vi "Main.vi"(10 "DAQ Type":enum16{"Hardware", "Simulation"}(ring), 11 "Module Admin":refnum<class "Delacor_lib_QMH_Module Admin.lvclass">) -> ()   [LabVIEW 2021, in "ARINC.lvlib"]
doc: "This template is based off of the Queued Message Handler design pattern and the Queued Message Handler project template that ships with LabVIEW.\n\nThe main difference is that the queue is private to this module and communication between modules is performed via Broadcast and Request events.\n\nRequest events are wrapped in public API methods and are handled in the Event Handling Loop (EHL) of this VI. Any module can register for Broadcast events sent by this module. The EHL generates messages based on user interface actions.\n\nThe Message Handling Loop (MHL) processes messages generated by the EHL, or by other messages. The messages are string values, so new messages can be added easily to the Message Cases case structure in the MHL. Each message cluster can also provide an optional value for Message Data, which is a variant that can be converted to whatever message-specific data is required.\n_____\nBased on DQMH Project Template 6.1.0.94."
uses:
  ARINC.lvlib
  <vilib>/Delacor/Delacor QMH/Libraries/Module Admin_class/Delacor_lib_QMH_Module Admin.lvclass
  Class/AIT 429/AIT 429.lvclass
  C:/repository/common_ATE/Libraries/ARINC/Class/Abstract/Abstract.lvclass
  Class/Abstract/Abstract.lvclass
  Module Data--cluster.ctl
  <vilib>/Delacor/Delacor QMH/Libraries/Message Queue_class/Delacor_lib_QMH_Message Queue.lvclass/Delacor_lib_QMH_Message Queue.ctl
  Stop Argument--cluster.ctl
  <vilib>/Delacor/Delacor QMH/Libraries/Module Admin_class/Delacor_lib_QMH_Module Admin.lvclass/Delacor_lib_QMH_Module Admin.ctl
  REQ Initialize Hardware Argument--cluster.ctl
  REQ Initialize Hardware (Reply Payload)--cluster.ctl
  REQ Close Ref Argument--cluster.ctl
  <vilib>/Utility/miscctls.llb/LVPointTypeDef.ctl
  <vilib>/Delacor/Delacor QMH/Libraries/Message Queue_class/Delacor_lib_QMH_Enqueue Message (Single).vi
  <vilib>/Delacor/Delacor QMH/Libraries/Module Admin_class/Delacor_lib_QMH_Get External Launch.vi
  <vilib>/Utility/error.llb/Error Cluster From Error Code.vi
  <vilib>/ErrorRing/Error Ring.xnode
  <vilib>/Delacor/Delacor QMH/Libraries/Message Queue_class/Delacor_lib_QMH_Message Queue.lvclass
panel:
  out "error out":errorcluster
  out "Status":string
  in  "Simulate MHL Error":bool
  in  "Simulate EHL Error":bool
  # "Other QMH Modules communicate with this Module via its Public API (wrappers for its Request Events).\n\nThis Module communicates with other Modules via its Broadcast Events.\nAny module that wants to get these messages, just registers for this module's Broadcast events."
  # "This template is for the Delacor Modified Queued Message Handler design pattern.\n\nSee the block diagram for more information on how to use this template."
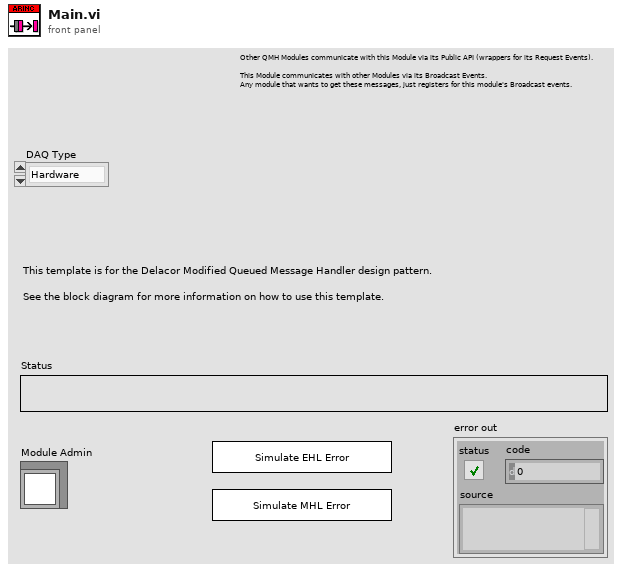
[diagram p1: front panel]
types:
  T1 = typedef "ARINC.lvlib/Request Events--cluster.ctl" = cluster{"Stop Module":refnum<user-event>, "Show Panel":refnum<user-event>, "Hide Panel":refnum<user-event>, "Get Module Execution Status":refnum<user-event>, "Show Diagram":refnum<user-event>, "REQ Initialize Hardware":refnum<user-event>, "REQ Close Ref":refnum<user-event>}
  T2 = typedef "ARINC.lvlib/Module Data--cluster.ctl" = cluster{"Status":string, "Abstract.lvclass":refnum<class "Abstract.lvclass">, "Connection Ref":variant}
  T3 = enum32{"invalid lock state", "Not Locked", "Locked (No Password)", "Password-protected"}
  T4 = typedef "ARINC.lvlib/Stop Argument--cluster.ctl" = cluster{"Origin":string, "Exit via Stop Module Req?":bool, "Wait for Module to stop?":bool}
  T5 = typedef "ARINC.lvlib/REQ Initialize Hardware Argument--cluster.ctl" = cluster{"Connection Ref":variant, "Wait Notifier":refnum<notifier>, "wait for reply":bool}
  T6 = typedef "ARINC.lvlib/REQ Close Ref Argument--cluster.ctl" = cluster{"Boolean":bool}
  T7 = typedef "LVPointTypeDef.ctl" = cluster{"Horizontal":i16, "Vertical":i16}
  T8 = enum32{"Invalid", "Standard", "Closed", "Hidden", "Minimized", "Maximized"}
  T9 = typedef "ARINC.lvlib/REQ Initialize Hardware (Reply Payload)--cluster.ctl" = cluster{"Connect?":bool, "error":errorcluster}
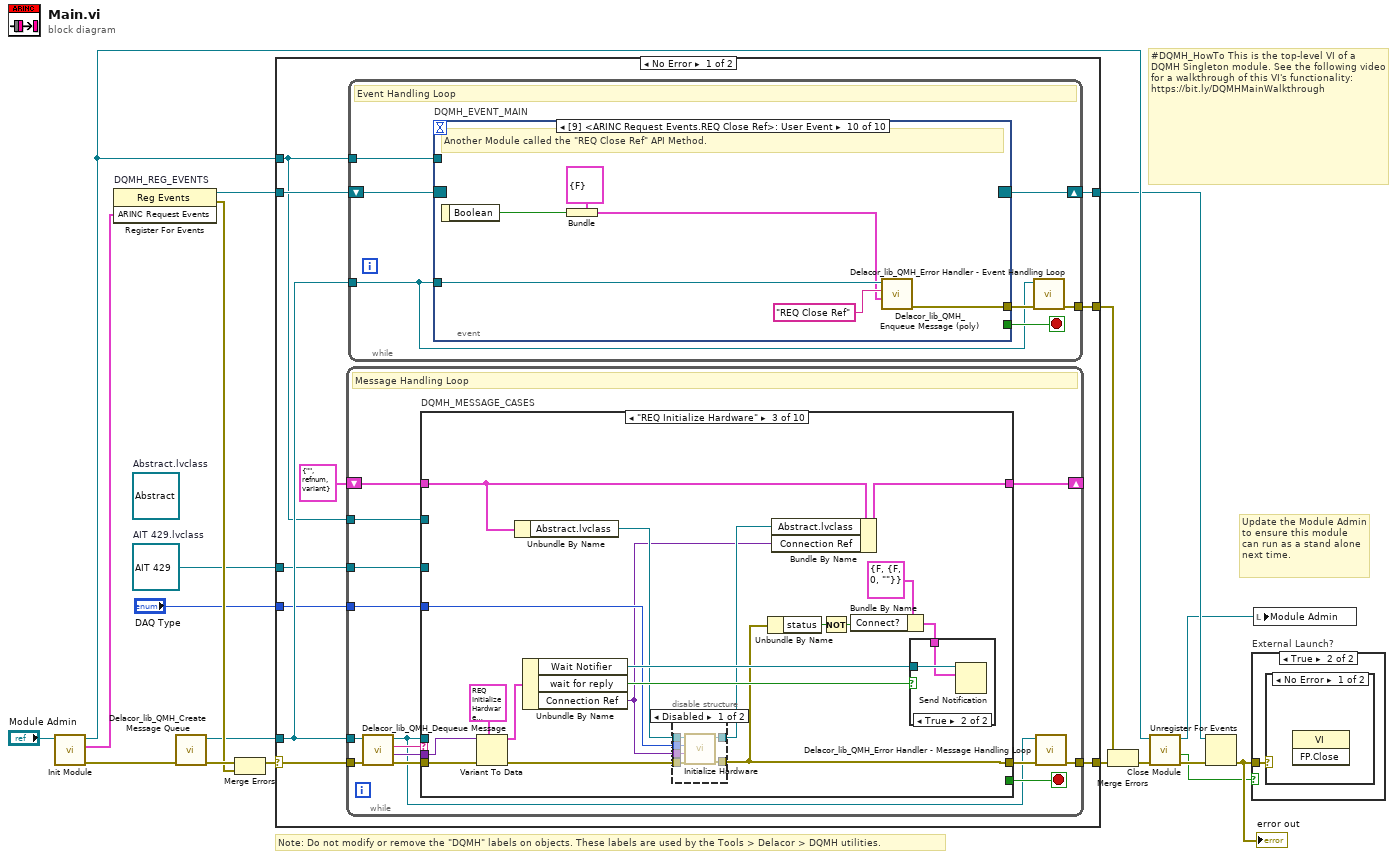
[diagram p0: block diagram]
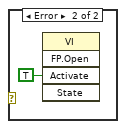
[diagram p3: hidden frame]
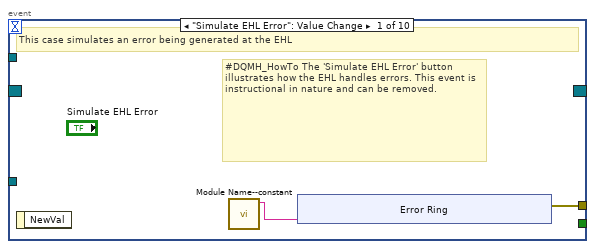
[diagram p4: hidden frame]
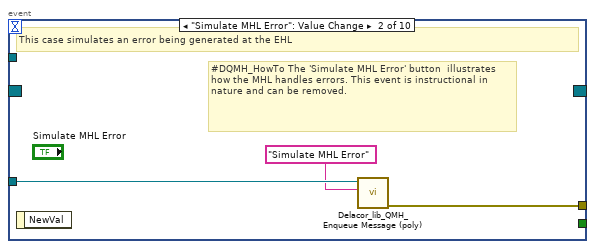
[diagram p5: hidden frame]
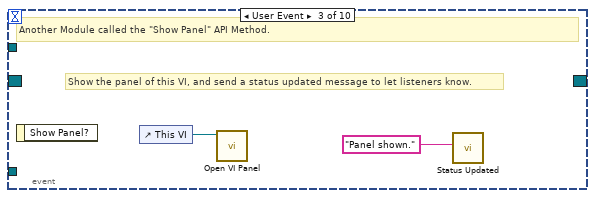
[diagram p6: hidden frame]
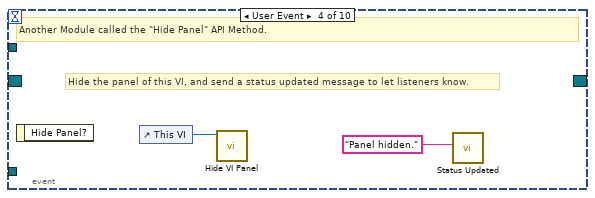
[diagram p7: hidden frame]
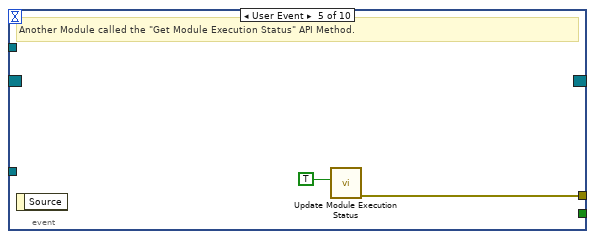
[diagram p8: hidden frame]
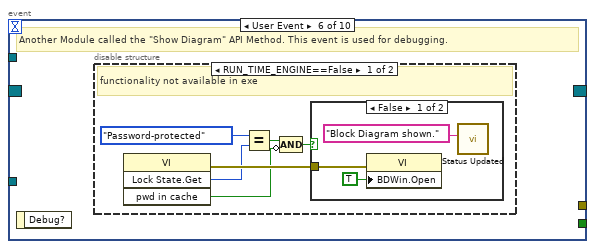
[diagram p9: hidden frame]
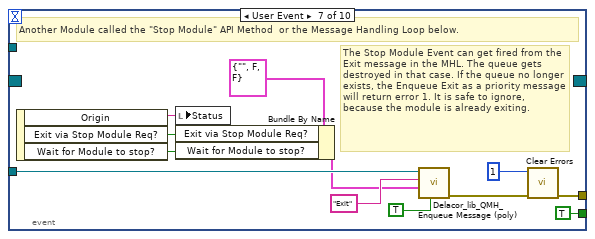
[diagram p12: hidden frame]
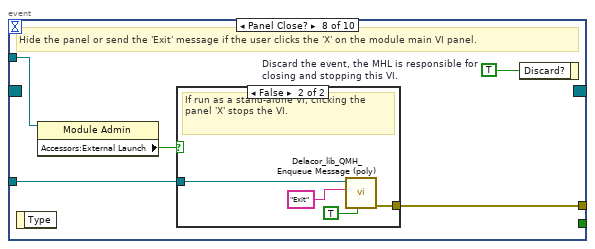
[diagram p13: hidden frame]
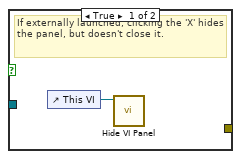
[diagram p14: hidden frame]
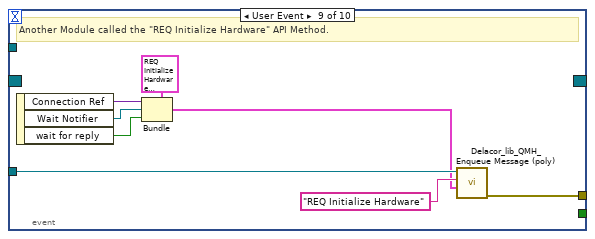
[diagram p15: hidden frame]
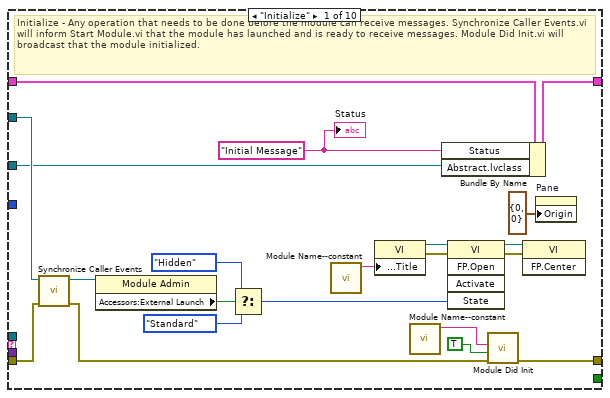
[diagram p16: hidden frame]
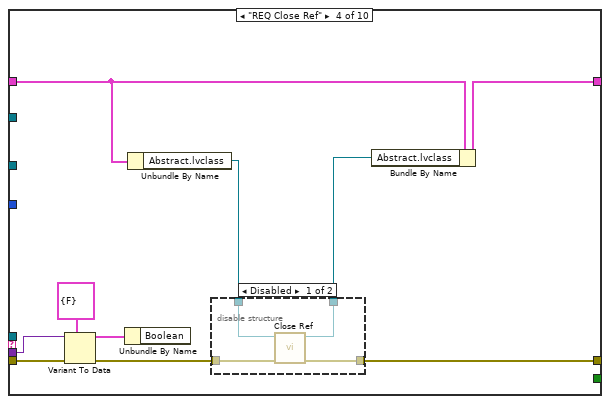
[diagram p20: hidden frame]
diagram:
  w2 = refnum<class "AIT 429.lvclass"> refnum  # AIT 429.lvclass
  (unwired) refnum<class "Abstract.lvclass"> refnum  # Abstract.lvclass
  # "#DQMH_HowTo This is the top-level VI of a DQMH Singleton module. See the following video for a walkthrough of this VI's functionality: https://bit.ly/DQMHMainWalkthrough"
  # "Note: Do not modify or remove the \"DQMH\" labels on objects. These labels are used by the Tools > Delacor > DQMH utilities."
  # "Update the Module Admin to ensure this module can run as a stand alone next time."
  n1 = call "Init Module.vi"("Singleton Module Admin in"="Module Admin") -> ("error out"=w18:errorcluster, "ARINC Request Events"=w7:T1, "Singleton Module Admin out"=w10:refnum<class "Delacor_lib_QMH_Module Admin.lvclass">)  [unwired: 8 in]
  n2 = register-events "DQMH_REG_EVENTS"(w7) -> (reference out=w8:refnum<event-registration>, error out=w11:errorcluster)  [unwired: 2 in]
  n3 = call <vilib>:"Delacor_lib_QMH_Create Message Queue.vi"("error in"=w18) -> ("error out"=w13:errorcluster, "Message Queue"=w6:refnum<class "Delacor_lib_QMH_Message Queue.lvclass">)  [unwired: 9 in]
  n4 = Merge Errors(w13, w11) -> (w12:errorcluster)
  n5 = case shown="No Error" w12 {
    selector: w12 -> [w27 w241]
    tunnel: [w29 w240] -> w19
    tunnel: [w26 w246] -> w9
    tunnel: w8 -> [w24 w246]
    tunnel: w6 -> [w23 w239]
    tunnel: [w28 _] -> w16
    tunnel: w10 -> [w22 w242]
    tunnel: w2 -> [w21 _]
    tunnel: "DAQ Type" -> [w20 _]
    frame No Error {
      n6 = while {
        tunnel: w23 -> [w104]
        shift-right: [w108] -> _
        shift-left: T2 {"Status"="", "Abstract.lvclass"=refnum, "Connection Ref"=variant} ("Data Cluster") -> [w109]
        tunnel: w27 -> [w112]
        tunnel: [w110] -> w29
        tunnel: w22 -> [w102]
        tunnel: w21 -> [w101]
        tunnel: w20 -> [w100]
        stop <- w107 stop-if-true
        # "Message Handling Loop"
        n7 = call-dynamic "Delacor_lib_QMH_Dequeue Message.vi"("error in"=w112, "Message Queue in"=w104) -> ("error out"=w111:errorcluster, "Message Data"=w105:variant, "Message"=w106:string, "Message Queue out"=w103:refnum<class "Delacor_lib_QMH_Message Queue.lvclass">)  [unwired: 6 in]
        n8 = case "DQMH_MESSAGE_CASES" shown="\"REQ Initialize Hardware\"" w106 {
          selector: w106 -> [_ _ _ _ _ _ _ _ _ w226]
          tunnel: w103 -> [_ _ _ _ _ _ _ w196 w218 _]
          tunnel: w111 -> [w132 w136 w154 w172 w179 w181 w186 w203 w224 w228]
          tunnel: [w130 w136 w139 w167 w178 w181 w185 w199 w221 w229] -> w113
          tunnel: w109 -> [w121 w135 w144 w166 w177 w180 w183 w198 w217 w227]
          tunnel: [w120 w135 w142 w164 w177 w180 w183 w198 w217 w227] -> w108
          tunnel: [_ _ _ _ _ _ _ _ w216 _] -> w107
          tunnel: w105 -> [_ _ w153 w171 _ _ _ w197 w215 _]
          tunnel: w102 -> [w122 _ _ _ _ _ _ w195 w210 _]
          tunnel: w101 -> [w114 _ _ _ _ _ _ _ _ _]
          tunnel: w100 -> [_ _ w145 _ _ _ _ _ _ _]
          frame "Initialize" {
            w116 = "Initial Message" ("Initial Message")
            # "Initialize - Any operation that needs to be done before the module can receive messages. Synchronize Caller Events.vi will inform Start Module.vi that the module has launched and is ready to receive messages. Module Did Init.vi will broadcast that the module initialized."
            n9 = call "Synchronize Caller Events.vi"("error in (no error)"=w132, "Singleton Module Admin in"=w122) -> ("error out"=w131:errorcluster, "Singleton Module Admin out"=w117:refnum<class "Delacor_lib_QMH_Module Admin.lvclass">)  [unwired: 8 in]
            n10 = property class="Module Admin"(reference=w117) -> ("Accessors:External Launch"=w126:bool)  [unwired: 1 in, 2 out]
            n11 = Select(t=T8."Hidden" ("State"), s=w126, f=T8."Standard" ("State")) -> (s? t:f=w123:T8)
            n12 = call "Module Name--constant.vi"() -> ("Module Name"=w129:string)  [unwired: 11 in]
            n13 = property class="VI"("Front Panel.Title"=w129) -> (reference out=w128:refnum<vi>, error out=w134:errorcluster)  [unwired: 2 in]
            n14 = call "Module Name--constant.vi"() -> ("Module Name"=w118:string)  [unwired: 11 in]
            n15 = Bundle By Name(cluster=w121, "Status"=w116, "Abstract.lvclass"=w114) -> (w120:T2)
            n16 = invoke class="VI" method="FP.Open"(reference=w128, error in=w134, "State"=w123) -> (reference out=w127:refnum<vi>, error out=w133:errorcluster)  [unwired: 2 in, 3 out]
            n17 = call "Module Did Init.vi"("error in (no error)"=w131, "Initialized?"=TRUE, "Origin"=w118) -> ("error out"=w130:errorcluster)  [unwired: 8 in]
            n18 = invoke class="VI" method="FP.Center"(reference=w127, error in=w133) -> ()  [unwired: 1 in, 3 out]
            n19 = property on="Pane" class="Pane"("Origin"=T7 {"Horizontal"=0, "Vertical"=0}) -> ()  [unwired: 2 in, 2 out]
            "Status" <- w116
          }
          frame "---Module Specific---" {
            # "Separator -- The following cases handle messages specific to this Module."
          }
          frame "REQ Initialize Hardware" {
            n20 = Variant To Data(error in=w154, type=T5 {"Connection Ref"=variant, "Wait Notifier"=refnum, "wait for reply"=FALSE} ("REQ Initialize Hardware Argument"), Variant=w153) -> (data=w151:T5, error out=w146:errorcluster)
            n21 = Unbundle By Name(w144) -> ("Abstract.lvclass"=w143:refnum<class "Abstract.lvclass">)
            n22 = Unbundle By Name(w151) -> ("Wait Notifier"=w150:refnum<notifier>, "wait for reply"=w149:bool, "Connection Ref"=w140:variant)
            n23 = disable-structure shown="Disabled" {
              disable-tunnel: w146 -> [w160 _]
              disable-tunnel: w145 -> [w159 _]
              disable-tunnel: w143 -> [w158 _]
              disable-tunnel: [w157 _] -> w141
              disable-tunnel: w140 -> [w156 _]
              disable-tunnel: [w155 _] -> w139
              frame Disabled {
                n24 = call-dynamic "Initialize Hardware.vi"("error in (no error)"=w160, "Connection Ref"=w156, "DAQ Type"=w159, "Abstract in"=w158) -> ("error out"=w155:errorcluster, "Abstract out"=w157:refnum<class "Abstract.lvclass">)  [unwired: 6 in]
              }
              frame Enabled {
              }
            }
            n25 = Unbundle By Name(w139) -> ("status"=w138:bool)
            n26 = Bundle By Name(cluster=w144, "Abstract.lvclass"=w141, "Connection Ref"=w140) -> (w142:T2)
            n27 = Not(x=w138) -> (.not. x?=w137:bool)
            n28 = Bundle By Name(cluster=T9 {"Connect?"=FALSE, "error"={"status"=FALSE, "code"=0, "source"=""}} ("REQ Initialize Hardware (Reply Payload)"), "Connect?"=w137) -> (w148:T9)
            n29 = case shown="True" w149 {
              tunnel: w150 -> [_ w162]
              tunnel: w148 -> [_ w161]
              frame False {
              }
              frame True {
                n30 = Send Notification(notification=w161, notifier=w162) -> ()  [unwired: 1 in, 2 out]
              }
            }
          }
          frame "REQ Close Ref" {
            n31 = Variant To Data(error in=w172, type=T6 {"Boolean"=FALSE} ("REQ Close Ref Argument"), Variant=w171) -> (data=w169:T6, error out=w168:errorcluster)
            n32 = Unbundle By Name(w169) -> ()  [unwired: 1 out]
            n33 = Unbundle By Name(w166) -> ("Abstract.lvclass"=w165:refnum<class "Abstract.lvclass">)
            n34 = disable-structure shown="Disabled" {
              disable-tunnel: w168 -> [w176 _]
              disable-tunnel: [w175 _] -> w167
              disable-tunnel: w165 -> [w174 _]
              disable-tunnel: [w173 _] -> w163
              frame Disabled {
                n35 = call-dynamic "Close Ref.vi"("error in (no error)"=w176, "Abstract in"=w174) -> ("error out"=w175:errorcluster, "Abstract out"=w173:refnum<class "Abstract.lvclass">)  [unwired: 8 in]
              }
              frame Enabled {
              }
            }
            n36 = Bundle By Name(cluster=w166, "Abstract.lvclass"=w163) -> (w164:T2)
          }
          frame "---Copy This Frame---" {
            # "Duplicate this frame when creating new messages.  Change this comment in the duplicated frame to describe this message."
            n37 = Merge Errors(w179) -> (w178:errorcluster)
          }
          frame "---Exit and Error Handling---" {
            # "Separator - The following cases handle errors and exit messages."
          }
          frame "Simulate MHL Error" {
            # "#DQMH_HowTo The 'Simulate MHL Error' button  illustrates how the MHL handles errors. This event is instructional in nature and can be removed."
            # "Simulate an error occurring at the MHL"
            n38 = call "Module Name--constant.vi"() -> ("Module Name"=w182:string)  [unwired: 11 in]
            n39 = xnode "Error Ring"("parameter 0"=w182) -> ("error out"=w184:errorcluster)
            n40 = Merge Errors(w186, w184) -> (w185:errorcluster)
          }
          frame "Error" {
            # "#CodeRecommended - If you ever change the name of this \"Error\" message, you'll need to update the name in the Check Loop Error.vi as well."
            # "#CodeRecommended - If the module is running in standalone mode (External Launch = FALSE), this code will pop up an error dialog and call the 'Exit' message if an error occurs. Add more fine-grained error handling here."
            # "Error - Check the error message data and respond accordingly. This message is sent by the \"Error Handler\" VIs at the end of each loop in this application."
            n41 = property class="Module Admin"(reference=w195) -> ("Accessors:External Launch"=w194:bool)  [unwired: 1 in, 2 out]
            n42 = Variant To Data(error in=w203, type=errorcluster {"status"=FALSE, "code"=0, "source"=""} ("error constant"), Variant=w197) -> (data=w204:errorcluster, error out=w201:errorcluster)
            n43 = call "Error Reported.vi"("Error"=w204) -> ()  [unwired: 10 in, 1 out]
            n44 = case shown="False" w194 {
              tunnel: [w209 _] -> w200
              tunnel: w196 -> [w207 _]
              tunnel: w204 -> [w208 _]
              frame False {
                # "If the module is running standalone, then pop up an error dialog and call the \"Exit\" message."
                n45 = call <vilib>:"Simple Error Handler.vi"("error in (no error)"=w208) -> ()  [unwired: 4 in, 5 out]
                n46 = call-poly <vilib>:"Delacor_lib_QMH_Enqueue Message (poly).vi"("Priority Message? (F)"=TRUE, "Message"="Exit", "Message Queue in"=w207) -> ("error out"=w209:errorcluster)  [unwired: 7 in, 1 out]
              }
              frame True {
                # "If the module was launched externally, calling the Error Reported broadcast VI is the only action performed by the \"Error\" message. The module's caller can then process the error appropriately."
              }
            }
            n47 = Merge Errors(w201, w200) -> (w199:errorcluster)
            n48 = local write "error out"(w199) -> ()
          }
          frame "Exit" {
            w214 = 91  # 91: not all Exit messages will have an argument
            w216 = TRUE  # Stop the VI
            # "Release the message queue reference"
            # "#CodeNeeded - Add any required cleanup code here"
            # "Exit - Exit the application."
            n49 = Variant To Data(error in=w224, type=T4 {"Origin"="", "Exit via Stop Module Req?"=FALSE, "Wait for Module to stop?"=FALSE} ("Stop Argument"), Variant=w215) -> (data=w212:T4, error out=w220:errorcluster)
            n50 = call <vilib>:"Clear Errors.vi"("error in (no error)"=w220, "specific error code to clear (0: all)"=w214) -> ("error out"=w223:errorcluster)  [unwired: 4 in, 1 out]
            n51 = control-ref of="This VI"() -> (w211:refnum<vi>)
            n52 = call-dynamic "Delacor_lib_QMH_Release Message Queue.vi"("error in"=w223, "Message Queue"=w218) -> ("error out"=w222:errorcluster)  [unwired: 9 in]
            n53 = call "Handle Exit.vi"("Stop Argument"=w212, "Admin in"=w210, "VI reference"=w211) -> ("error out"=w219:errorcluster)  [unwired: 7 in, 1 out]
            n54 = Merge Errors(w222, w219) -> (w221:errorcluster)
          }
          frame Default {
            # "'Default' case only runs if there is a message that isn't defined in any of the other cases.  Output a programming error."
            n55 = call "Module Name--constant.vi"() -> ("Module Name"=w225:string)  [unwired: 11 in]
            n56 = xnode "Error Ring"("parameter 0"=w226, "parameter 1"=w225) -> ("error out"=w230:errorcluster)
            n57 = Merge Errors(w228, w230) -> (w229:errorcluster)
          }
        }
        n58 = call-dynamic "Delacor_lib_QMH_Error Handler - Message Handling Loop.vi"("error in"=w113, "Message Queue in"=w103) -> ("dup error in"=w110:errorcluster)  [unwired: 8 in, 1 out]
      }
      n59 = while {
        tunnel: w23 -> [w30]
        shift-right: [w33] -> w26
        shift-left: w24 -> [w34]
        tunnel: [w35] -> w28
        tunnel: w22 -> [w31]
        stop <- w32 stop-if-true
        # "Event Handling Loop"
        n60 = event "DQMH_EVENT_MAIN" shown="[9] <ARINC Request Events.REQ Close Ref>: User Event" {
          selector: w34 -> [_ _ _ _ _ _ _ _ _ _]
          dyn-events: [_ _ _ _ _ _ _ _ _ _] -> w33
          timeout: _ -> [_ _ _ _ _ _ _ _ _ _]
          tunnel: [_ _ _ _ _ _ TRUE ("Discard?") _ _ _] -> w32
          tunnel: w30 -> [_ w47 _ _ _ _ w71 w78 w93 w99]
          tunnel: [w38 w48 _ _ w54 _ w74 w80 w86 w94] -> w36
          tunnel: w31 -> [_ _ _ _ _ _ _ w77 _ _]
          event "Simulate EHL Error": Value Change {
            # "#DQMH_HowTo The 'Simulate EHL Error' button  illustrates how the EHL handles errors. This event is instructional in nature and can be removed."
            # "This case simulates an error being generated at the EHL"
            n61 = event-data() -> ()  [unwired: 1 in, 1 out]
            n62 = call "Module Name--constant.vi"() -> ("Module Name"=w37:string)  [unwired: 11 in]
            n63 = xnode "Error Ring"("parameter 0"=w37) -> ("error out"=w38:errorcluster)
          }
          event "Simulate MHL Error": Value Change {
            # "#DQMH_HowTo The 'Simulate MHL Error' button  illustrates how the MHL handles errors. This event is instructional in nature and can be removed."
            # "This case simulates an error being generated at the EHL"
            n64 = event-data() -> ()  [unwired: 1 in, 1 out]
            n65 = call-poly <vilib>:"Delacor_lib_QMH_Enqueue Message (poly).vi"("Message"="Simulate MHL Error", "Message Queue in"=w47) -> ("error out"=w48:errorcluster)  [unwired: 8 in, 1 out]
          }
          event User Event {
            # "Show the panel of this VI, and send a status updated message to let listeners know."
            # "Another Module called the \"Show Panel\" API Method."
            n66 = event-data() -> ()  [unwired: 1 in, 1 out]
            n67 = control-ref of="This VI"() -> (w50:refnum<vi>)
            n68 = call "Open VI Panel.vi"("VI"=w50) -> ()  [unwired: 10 in, 1 out]
            n69 = call "Status Updated.vi"("Status"="Panel shown." ("format string")) -> ()  [unwired: 10 in, 1 out]
          }
          event User Event {
            # "Hide the panel of this VI, and send a status updated message to let listeners know."
            # "Another Module called the \"Hide Panel\" API Method."
            n70 = event-data() -> ()  [unwired: 1 in, 1 out]
            n71 = control-ref of="This VI"() -> (w52:refnum<vi>)
            n72 = call "Hide VI Panel.vi"("VI"=w52) -> ()  [unwired: 10 in, 1 out]
            n73 = call "Status Updated.vi"("Status"="Panel hidden." ("format string")) -> ()  [unwired: 10 in, 1 out]
          }
          event User Event {
            # "Another Module called the \"Get Module Execution Status\" API Method."
            n74 = event-data() -> ()  [unwired: 1 in, 1 out]
            n75 = call "Update Module Execution Status.vi"("Running?"=TRUE) -> ("error out"=w54:errorcluster)  [unwired: 10 in]
          }
          event User Event {
            # "Another Module called the \"Show Diagram\" API Method. This event is used for debugging."
            n76 = event-data() -> ()  [unwired: 1 in, 1 out]
            n77 = disable-structure shown="RUN_TIME_ENGINE==False" {
              frame condition #0 (active) {
                # "functionality not available in exe"
                n78 = invoke class="VI" method="Lock State.Get"() -> (error out=w60:errorcluster, "Get Lock State"=w59:T3, "pwd in cache"=w56:bool)  [unwired: 4 in, 1 out]
                n79 = Equal?(x=T3."Password-protected", y=w59) -> (x = y?=w57:bool)
                n80 = Compound Arithmetic op=AND(w57, invert w56) -> (w55:bool)
                n81 = case shown="False" w55 {
                  tunnel: w60 -> [w63 _]
                  frame False {
                    n82 = property class="VI"(error in=w63, "BDWin.Open"=TRUE ("Block Diagram Window:Open")) -> ()  [unwired: 1 in, 2 out]
                    n83 = call "Status Updated.vi"("Status"="Block Diagram shown." ("format string")) -> ()  [unwired: 10 in, 1 out]
                  }
                  frame True {
                    # "Password-protected VI, and the password is not in the cache. Do not show the diagram."
                  }
                }
              }
              frame condition #1 {
              }
            }
          }
          event User Event {
            # "The Stop Module Event can get fired from the Exit message in the MHL. The queue gets destroyed in that case. If the queue no longer exists, the Enqueue Exit as a priority message will return error 1. It is safe to ignore, because the module is already exiting."
            # "Another Module called the \"Stop Module\" API Method  or the Message Handling Loop below."
            n84 = event-data() -> ("Origin"=w70:string, "Exit via Stop Module Req?"=w66:bool, "Wait for Module to stop?"=w65:bool)  [unwired: 1 in]
            n85 = local write "Status"(w70) -> ()
            n86 = Bundle By Name(cluster=T4 {"Origin"="", "Exit via Stop Module Req?"=FALSE, "Wait for Module to stop?"=FALSE} ("Stop Argument"), "Exit via Stop Module Req?"=w66, "Wait for Module to stop?"=w65) -> (w64:T4)
            n87 = call-poly <vilib>:"Delacor_lib_QMH_Enqueue Message (poly).vi"("Priority Message? (F)"=TRUE, "Message Data"=w64, "Message"="Exit", "Message Queue in"=w71) -> ("error out"=w75:errorcluster)  [unwired: 6 in, 1 out]
            n88 = call <vilib>:"Clear Errors.vi"("error in (no error)"=w75, "specific error code to clear (0: all)"=1) -> ("error out"=w74:errorcluster)  [unwired: 4 in, 1 out]
          }
          event Panel Close? {
            w79 = TRUE  # Discard the event, the MHL is responsible for closing and stopping this VI.
            # "Hide the panel or send the 'Exit' message if the user clicks the 'X' on the module main VI panel."
            n89 = event-data() -> ()  [unwired: 1 in, 1 out]
            n90 = property class="Module Admin"(reference=w77) -> ("Accessors:External Launch"=w76:bool)  [unwired: 1 in, 2 out]
            n91 = case shown="False" w76 {
              tunnel: w78 -> [_ w84]
              tunnel: [_ w85] -> w80
              frame True {
                # "If externally launched, clicking the 'X' hides the panel, but doesn't close it."
                n92 = control-ref of="This VI"() -> (w81:refnum<vi>)
                n93 = call "Hide VI Panel.vi"("VI"=w81) -> ()  [unwired: 10 in, 1 out]
              }
              frame False {
                # "If run as a stand-alone VI, clicking the panel 'X' stops the VI."
                n94 = call-poly <vilib>:"Delacor_lib_QMH_Enqueue Message (poly).vi"("Priority Message? (F)"=TRUE, "Message"="Exit", "Message Queue in"=w84) -> ("error out"=w85:errorcluster)  [unwired: 7 in, 1 out]
              }
            }
            n95 = event-data("Discard?"=w79) -> ()  [unwired: 1 in, 1 out]
          }
          event User Event {
            # "Another Module called the \"REQ Initialize Hardware\" API Method."
            n96 = event-data() -> ("Connection Ref"=w89:variant, "Wait Notifier"=w88:refnum<notifier>, "wait for reply"=w87:bool)  [unwired: 1 in]
            n97 = Bundle(cluster=T5 {"Connection Ref"=variant, "Wait Notifier"=refnum, "wait for reply"=FALSE} ("REQ Initialize Hardware Argument"), "Connection Ref"=w89, "Wait Notifier"=w88, "wait for reply"=w87) -> (w90:T5)
            n98 = call-poly <vilib>:"Delacor_lib_QMH_Enqueue Message (poly).vi"("Message Data"=w90, "Message"="REQ Initialize Hardware", "Message Queue in"=w93) -> ("error out"=w86:errorcluster)  [unwired: 7 in, 1 out]
          }
          event User Event {
            # "Another Module called the \"REQ Close Ref\" API Method."
            n99 = event-data() -> ("Boolean"=w95:bool)  [unwired: 1 in]
            n100 = Bundle(cluster=T6 {"Boolean"=FALSE} ("REQ Close Ref Argument"), "Boolean"=w95) -> (w96:T6)
            n101 = call-poly <vilib>:"Delacor_lib_QMH_Enqueue Message (poly).vi"("Message Data"=w96, "Message"="REQ Close Ref", "Message Queue in"=w99) -> ("error out"=w94:errorcluster)  [unwired: 7 in, 1 out]
          }
        }
        n102 = call-dynamic "Delacor_lib_QMH_Error Handler - Event Handling Loop.vi"("error in"=w36, "Message Queue in"=w30) -> ("dup error in"=w35:errorcluster)  [unwired: 8 in, 1 out]
      }
    }
    frame Error {
      # "Synchronize Caller Events.vi will inform Start Module.vi that the module has launched and will let the code calling Start Module.vi register for broadcasts and would permit the caller receive the broadcast that an error occurred at launch time."
      n103 = call-dynamic "Delacor_lib_QMH_Release Message Queue.vi"("error in"=w241, "Message Queue"=w239) -> ("error out"=w240:errorcluster)  [unwired: 9 in]
      n104 = call "Synchronize Caller Events.vi"("Singleton Module Admin in"=w242) -> ("error out"=w247:errorcluster)  [unwired: 9 in, 1 out]
      n105 = call "Module Name--constant.vi"() -> ("Module Name"=w245:string)  [unwired: 11 in]
      n106 = Format Into String(format string="An error occurred during initialization. %s is no longer running.", w245) -> (resulting string=w243:string)  [unwired: 2 in, 1 out]
      n107 = Merge Errors(w240, w247) -> (w248:errorcluster)
      n108 = call "Error Reported.vi"("Additional Information"=w243, "Error"=w248) -> ()  [unwired: 9 in, 1 out]
    }
  }
  n109 = Merge Errors(w16, w19) -> (w15:errorcluster)
  n110 = call "Close Module.vi"("error in (no error)"=w15, "Module Admin in"=w10) -> ("error out"=w17:errorcluster, "External Launch"=w3:bool, "Module Admin out"=w4:refnum<class "Delacor_lib_QMH_Module Admin.lvclass">)  [unwired: 7 in]
  n111 = Unregister For Events(event registration refnum=w9, error in=w17) -> (error out=w14:errorcluster)
  "error out" <- w14
  n112 = case "External Launch?" shown="True" w3 {
    tunnel: w14 -> [_ w249]
    frame False {
    }
    frame True {
      n113 = case shown="No Error" w249 {
        frame No Error {
          n114 = invoke class="VI" method="FP.Close"() -> ()  [unwired: 3 in, 3 out]
        }
        frame Error {
          n115 = invoke class="VI" method="FP.Open"("Activate"=TRUE ("Activate?")) -> ()  [unwired: 4 in, 5 out]
        }
      }
    }
  }
  n116 = local write "Module Admin"(w4) -> ()
